vi "Change Control Size.vi"(8 "error in (no error)":errorcluster, 9 "dSize":cluster{"Width":i32, "Height":i32}, 11 "Ctl Refnum":refnum<vi>) -> (0 "error out":errorcluster, 2 "changed?":bool, 3 "refnum dub":refnum<vi>)   [LabVIEW 2014, in "POLARIS Vision utility.lvlib"]
uses:
  POLARIS Vision utility.lvlib
  XDisplay/POLARIS IMAQ Display.xctl
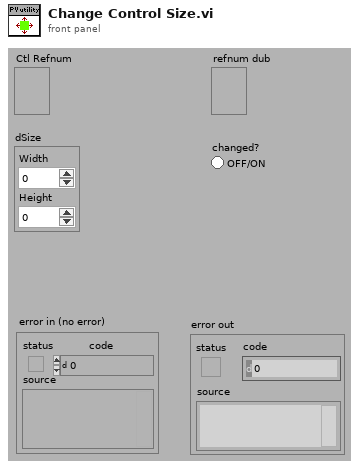
[diagram p1: front panel]
types:
  T1 = typedef "LVBoundsTypeDef.ctl" = cluster{"Width":u32, "Height":u32}
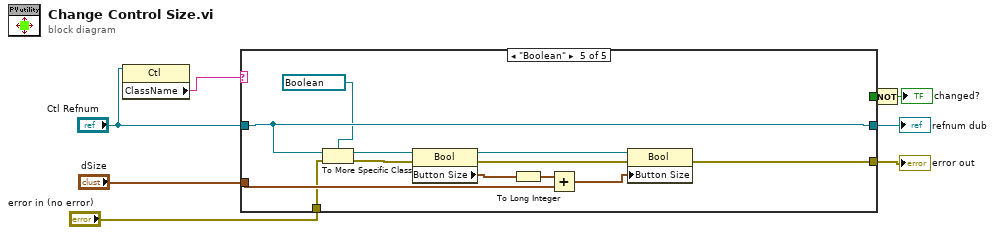
[diagram p0: block diagram]
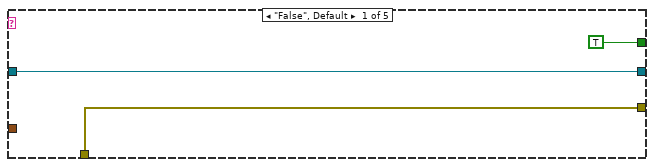
[diagram p2: hidden frame]
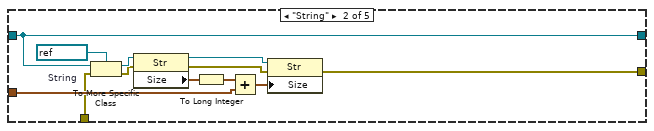
[diagram p3: hidden frame]
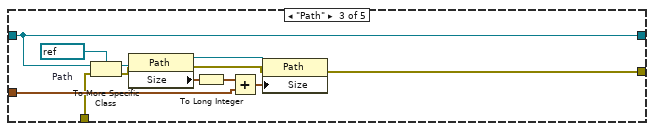
[diagram p4: hidden frame]
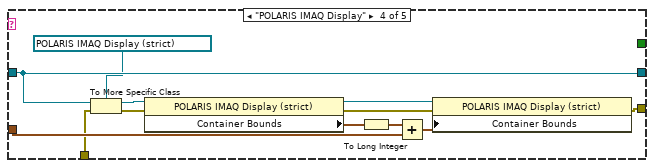
[diagram p5: hidden frame]
diagram:
  n1 = property class="Ctl"(reference="Ctl Refnum") -> ("ClassName"=w1:string)  [unwired: 1 in, 2 out]
  n2 = case shown="\"Boolean\"" w1 {
    tunnel: [w11 w13 w24 w42 w56] -> w7
    tunnel: "Ctl Refnum" -> [w11 w13 w24 w42 w56]
    tunnel: "dSize" -> [_ w17 w29 w41 w58]
    tunnel: "error in (no error)" -> [w10 w16 w28 w40 w57]
    tunnel: [w10 w12 w25 w37 w50] -> w5
    tunnel: [TRUE _ _ _ _] -> w4
    frame "False", Default {
    }
    frame "String" {
      w22 = refnum<vi> refnum  # String
      n3 = To More Specific Class(target class=w22, reference=w13, error in=w16) -> (specific class reference=w23:refnum<vi>, error out=w15:errorcluster)
      n4 = property class="Str"(reference=w23, error in=w15) -> (reference out=w21:refnum<vi>, error out=w14:errorcluster, "Size"=w20:T1)
      n5 = To Long Integer(number=w20) -> (32bit integer=w18:cluster{"Width":i32, "Height":i32})
      n6 = Add(x=w18, y=w17) -> (x+y=w19:cluster{"Width":i32, "Height":i32})
      n7 = property class="Str"(reference=w21, error in=w14, "Size"=w19) -> (error out=w12:errorcluster)  [unwired: 1 out]
    }
    frame "Path" {
      w34 = refnum<vi> refnum  # Path
      n8 = To More Specific Class(target class=w34, reference=w24, error in=w28) -> (specific class reference=w35:refnum<vi>, error out=w27:errorcluster)
      n9 = property class="Path"(reference=w35, error in=w27) -> (reference out=w33:refnum<vi>, error out=w26:errorcluster, "Size"=w32:T1)
      n10 = To Long Integer(number=w32) -> (32bit integer=w30:cluster{"Width":i32, "Height":i32})
      n11 = Add(x=w30, y=w29) -> (x+y=w31:cluster{"Width":i32, "Height":i32})
      n12 = property class="Path"(reference=w33, error in=w26, "Size"=w31) -> (error out=w25:errorcluster)  [unwired: 1 out]
    }
    frame "POLARIS IMAQ Display" {
      n13 = To More Specific Class(target class=refnum<vi> refnum ("POLARIS IMAQ"), reference=w42, error in=w40) -> (specific class reference=w47:refnum<vi>, error out=w39:errorcluster)
      n14 = property class="POLARIS IMAQ Display (strict)"(reference=w47, error in=w39) -> (reference out=w46:refnum<vi>, error out=w38:errorcluster, "Container Bounds"=w45:T1)
      n15 = To Long Integer(number=w45) -> (32bit integer=w43:cluster{"Width":i32, "Height":i32})
      n16 = Add(x=w43, y=w41) -> (x+y=w44:cluster{"Width":i32, "Height":i32})
      n17 = property class="POLARIS IMAQ Display (strict)"(reference=w46, error in=w38, "Container Bounds"=w44) -> (error out=w37:errorcluster)  [unwired: 1 out]
    }
    frame "Boolean" {
      n18 = To More Specific Class(target class=refnum<vi> refnum ("Bool Refnum"), reference=w56, error in=w57) -> (specific class reference=w55:refnum<vi>, error out=w54:errorcluster)
      n19 = property class="Bool"(reference=w55, error in=w54) -> (reference out=w51:refnum<vi>, error out=w49:errorcluster, "Button Size"=w52:T1)
      n20 = To Long Integer(number=w52) -> (32bit integer=w59:cluster{"Width":i32, "Height":i32})
      n21 = Add(x=w59, y=w58) -> (x+y=w53:cluster{"Width":i32, "Height":i32})
      n22 = property class="Bool"(reference=w51, error in=w49, "Button Size"=w53) -> (error out=w50:errorcluster)  [unwired: 1 out]
    }
  }
  "refnum dub" <- w7
  "error out" <- w5
  n23 = Not(x=w4) -> (.not. x?=→"changed?":bool)
